vi "Tell Self.vi"(4 "Priority":bool, 10 "Msg":refnum<class "Msg.lvclass">, 11 "Core Actor in":refnum<class "Core Actor.lvclass">) -> (0 "Error out":errorcluster)   [LabVIEW 2025, in "jettl.lvlib" / "Core Actor.lvlib" / "Core Actor.lvclass"]
uses:
  Core Actor.lvclass
  Msg/Msg.lvclass
  Relation.ctl
  Attributes/Attributes/Attributes.lvclass
  Transport/Transport/Transport.lvclass
  Core Actor.lvclass/Core Actor.ctl
  jettl.lvlib
  Error/Error.lvlib
  Teller/Teller.lvlib
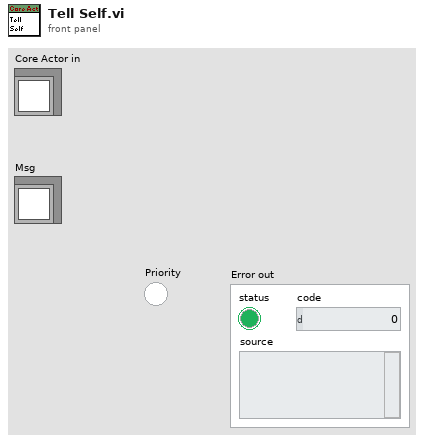
[diagram p1: front panel]
types:
  T1 = typedef "jettl.lvlib/Msg Set.ctl" = set{refnum<class "Msg.lvclass">}
  T2 = typedef "jettl.lvlib/Relation.ctl" = enum16{"Self", "Parent", "Child"}
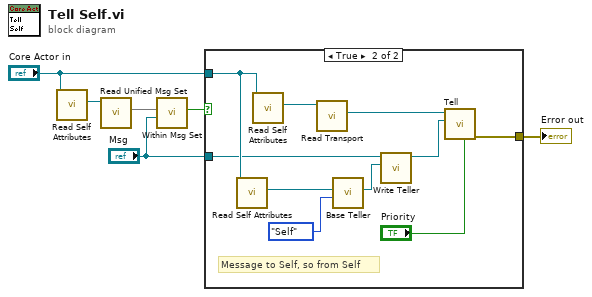
[diagram p0: block diagram]
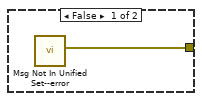
[diagram p2: hidden frame]
diagram:
  n1 = call-dynamic "Read Self Attributes.vi"("Core Actor in"="Core Actor in") -> ("Self Attributes"=w3:refnum<class "Attributes.lvclass">)  [unwired: 10 in]
  n2 = call-dynamic "Read Unified Msg Set.vi"("Attributes in"=w3) -> ("Unified Msg Set"=w2:T1)  [unwired: 10 in]
  n3 = call "Within Msg Set.vi"("Msg"="Msg", "Msg Set"=w2) -> ("Within Msg Set"=w6:bool)  [unwired: 9 in]
  n4 = case shown="True" w6 {
    tunnel: "Core Actor in" -> [_ w17]
    tunnel: "Msg" -> [_ w14]
    tunnel: [w7 w8] -> w1
    frame False {
      n5 = call "Msg Not In Unified Set--error.vi"() -> ("Error"=w7:errorcluster)  [unwired: 11 in]
    }
    frame True {
      # "Message to Self, so from Self"
      n6 = call-dynamic "Read Self Attributes.vi"("Core Actor in"=w17) -> ("Self Attributes"=w13:refnum<class "Attributes.lvclass">)  [unwired: 10 in]
      n7 = call-dynamic "Read Self Attributes.vi"("Core Actor in"=w17) -> ("Self Attributes"=w16:refnum<class "Attributes.lvclass">)  [unwired: 10 in]
      n8 = call-dynamic "Read Transport.vi"("Attributes in"=w16) -> ("Transport"=w11:refnum<class "Transport.lvclass">)  [unwired: 10 in]
      n9 = call "Base Teller.vi"("Relation"=Relation."Self", "Self Attributes"=w13) -> ("Teller"=w15:refnum<class "Teller.lvclass">)  [unwired: 9 in]
      n10 = call-dynamic "Write Teller.vi"("Teller"=w15, "Msg in"=w14) -> ("Msg out"=w10:refnum<class "Msg.lvclass">)  [unwired: 9 in]
      n11 = call-dynamic "Tell.vi"("Priority"="Priority", "Msg"=w10, "Transport in"=w11) -> ("Error out"=w8:errorcluster)  [unwired: 8 in]
    }
  }
  "Error out" <- w1
